vi "Initialize.vi"(0 "instance":u8) -> (4 "subsystem":refnum<class "Single Address Space Collection.lvclass">, 6 "AddressSpace":refnum<class "AddressSpace.lvclass">)   [LabVIEW 2017, in "BuckBoost.lvlib" / "AddressSpace.lvclass"]
uses:
  AddressSpace.lvclass
  <instrlib>/_niInstr/Instruction Framework/v1/FPGA/Helper Classes/Single Address Space Collection/Single Address Space Collection.lvclass
  C:/Program Files (x86)/National Instruments/LabVIEW 2017/instr.lib/_niInstr/Instruction Framework/v1/FPGA/Interfaces/Address Space/Address Space.lvclass
  AddressSpace.lvclass/AddressSpace.ctl
  <vilib>/rvi/eio/common/nirviEmuReportErrorAndStop.vi
  <vilib>/rvi/DataTransferAndStorage/Container/Common/niFpgaContainerSetEmuInfo.vi
  <vilib>/rvi/DataTransferAndStorage/Container/Common/niFpgaContainerGetUniqueNameForEmu.vi
  <vilib>/rvi/LocalResourceManager/LocalResourceManager.xnode
  BuckBoost.lvlib
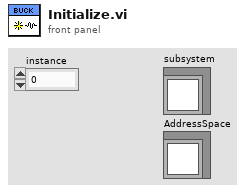
[diagram p1: front panel]
types:
  T1 = typedef "BuckBoost.lvlib/modRegisters.ctl" = cluster{"numberOfInterleaves":refnum<k21>, "Enable":refnum<k21>, "triangleInc":refnum<k21>, "Deadband":refnum<k21>, "Enabled":refnum<k21>}
  T2 = typedef "BuckBoost.lvlib/contSettings.ctl" = cluster{"numberOfInterleaves":refnum<k21>, "rampRate":refnum<k21>, "manualInput":refnum<k21>, "perturbAmp":refnum<k21>, "perturbAngleInc":refnum<k21>, "reset":refnum<k21>, "state":refnum<k21>, "gains":refnum<k21>, "Currents":refnum<k21>}
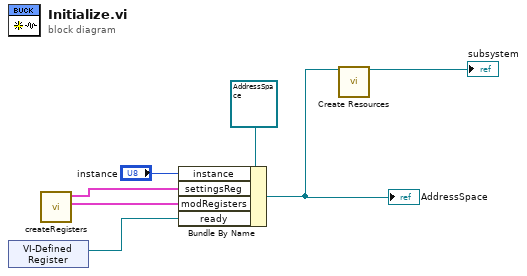
[diagram p0: block diagram]
diagram:
  n1 = xnode "VI-Defined Register"() -> ("Register Out"=w3:refnum<k21>)
  n2 = call "createRegisters.vi"() -> ("modRegisters"=w4:T1, "settingsReg"=w5:T2)  [unwired: 10 in]
  n3 = Bundle By Name(cluster=refnum<class "AddressSpace.lvclass"> refnum ("BuckBoost.lvlib:AddressSpace.lvclass"), "instance"="instance", "settingsReg"=w5, "modRegisters"=w4, "ready"=w3) -> (w2:refnum<class "AddressSpace.lvclass">)
  "AddressSpace" <- w2
  n4 = call <instrlib>:"Create Resources.vi"("address space"=w2) -> ("single address space collection"=→"subsystem":refnum<class "Single Address Space Collection.lvclass">)  [unwired: 14 in]
